vi "Create Container.vi"(8 "Error In":errorcluster, 11 "MDI Area Builder in":refnum<class "MDI Area Builder.lvclass">) -> (0 "Error Out":errorcluster, 2 "Container":refnum<class "QWidget.lvclass">, 3 "MDI Area Builder out":refnum<class "MDI Area Builder.lvclass">)   [LabVIEW 2013, in "MDI Area Builder.lvclass"]
uses:
  MDI Area Builder.lvclass
  src/LabVIEW/Qt Widgets/QWidget/QWidget.lvclass
  src/LabVIEW/LQ Core/Qt/ScrollBarPolicy.ctl
  src/LabVIEW/Qt Widgets/QAbstractScrollArea/setHorizontalScrollBarPolicy.vi
  src/LabVIEW/Qt Widgets/QAbstractScrollArea/setVerticalScrollBarPolicy.vi
  src/LabVIEW/Qt Widgets/QMdiArea/QMdiArea.lvclass
  src/LabVIEW/LQ Core/Qt/Qt.lvlib
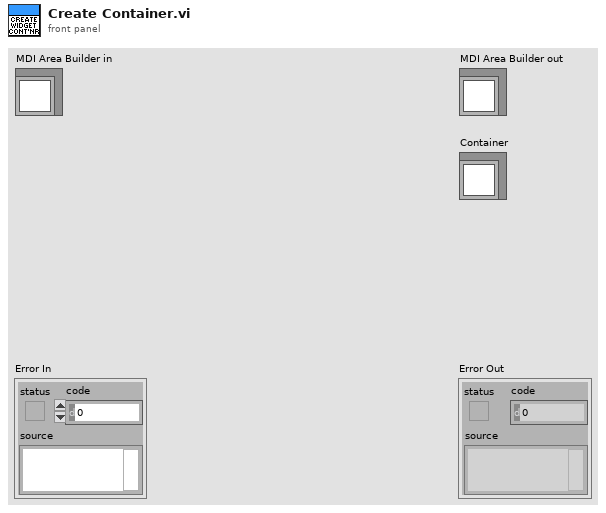
[diagram p1: front panel]
types:
  T1 = typedef "Qt.lvlib/ScrollBarPolicy.ctl" = i32
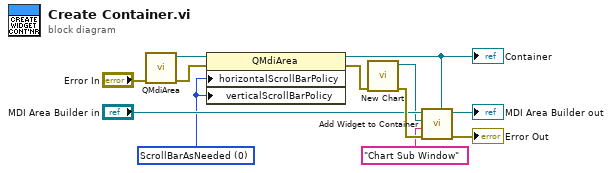
[diagram p0: block diagram]
diagram:
  w5 = T1 0 items=["ScrollBarAsNeeded", "ScrollBarAlwaysOff", "ScrollBarAlwaysOn"] ("horizontalScrollBarPolicy")
  n1 = call "QMdiArea.vi"("Error In"="Error In") -> ("Error Out"=w2:errorcluster, "New QMdiArea"=w4:refnum<class "QMdiArea.lvclass">)  [unwired: 9 in]
  n2 = property class="QMdiArea"(reference=w4, error in=w2, "horizontalScrollBarPolicy"=w5, "verticalScrollBarPolicy"=w5) -> (reference out=w3:refnum<class "QMdiArea.lvclass">, error out=w1:errorcluster)
  "Container" <- w3
  n3 = call "New Chart.vi"("Error In"=w1) -> ("Error Out"=w12:errorcluster, "New LQChart"=w7:refnum<class "LQChart.lvclass">)  [unwired: 9 in]
  n4 = call-dynamic "Add Widget to Container.vi"("Container"=w3, "Error In"=w12, "Label"="Chart Sub Window" ("windowTitle"), "Widget"=w7, "MDI Area Builder in"="MDI Area Builder in") -> ("Error Out"=→"Error Out":errorcluster, "MDI Area Builder out"=→"MDI Area Builder out":refnum<class "MDI Area Builder.lvclass">)  [unwired: 5 in]
